vi "Get INFO from ini FILE - AMSClient.vi"(0 "ini Name":string="AMSClient.ini", 5 "Application Directory (Default if blank)":path, 11 "Error In":errorcluster) -> (1 "Settings":T3, 4 "ini Path":path=path "C:/Users/CK/workspace/LabVIEW/Configuration File Test/MyEXE.ini", 6 "Connection Information":T1={"Connection "="SQL Server 32bit HPEnvy", "Username"="admin", "Password"="admin123"}, 8 "AMS Connection Information":T1={"Connection "="SQL Server 32bit HPEnvy", "Username"="admin", "Password"="admin123"}, 10 "Settings Boolean":T2, 12 "MessageQ":string, 15 "Error Out":errorcluster)   [LabVIEW 2013]
uses:
  Controls/Connection Information Cluster.ctl
  <vilib>/Utility/config.llb/Read Key (String).vi
  <vilib>/Utility/config.llb/Read Key (Boolean).vi
  <vilib>/Utility/config.llb/NI_LVConfig.lvlib
  <vilib>/Utility/config.llb/Write Key (I32).vi
panel:
  out "Application Directory":path=path "C:/Users/CK/workspace/LabVIEW/Configuration File Test"
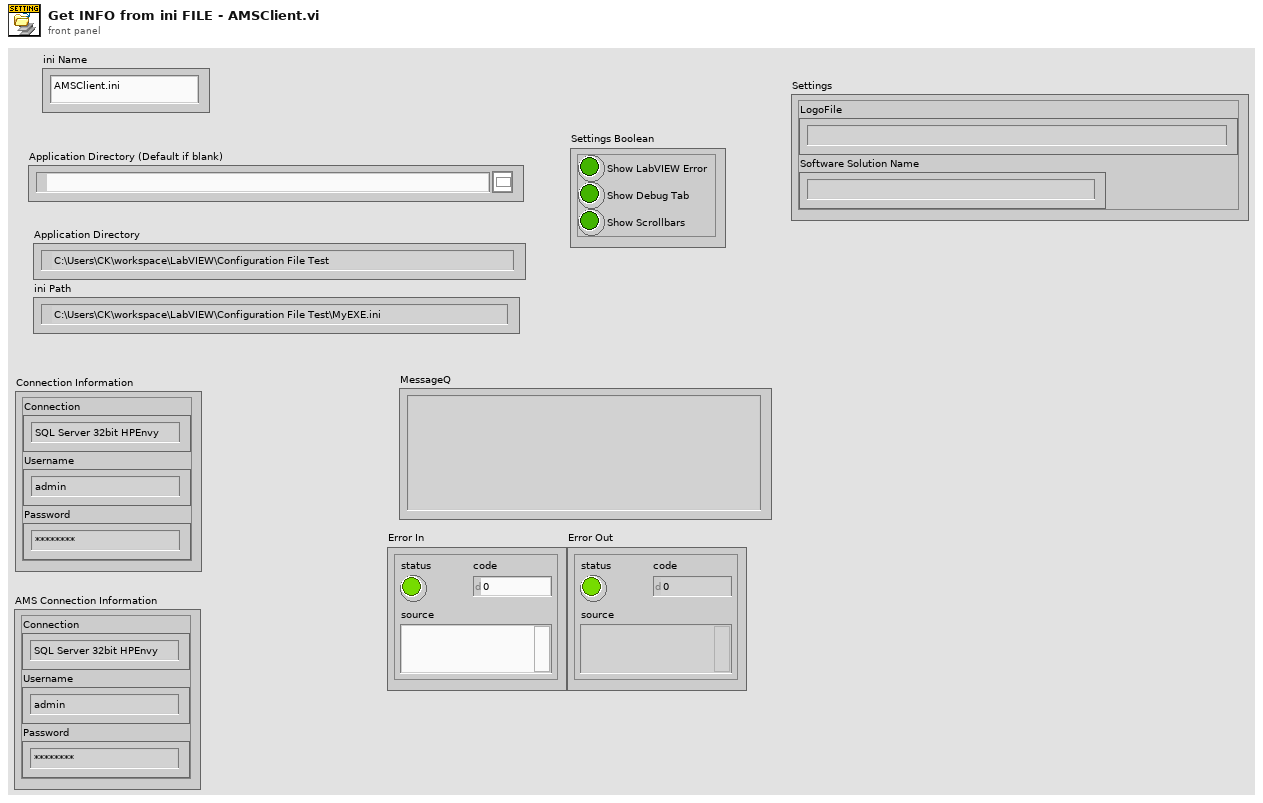
[diagram p1: front panel]
types:
  T1 = typedef "Connection Information Cluster.ctl" = cluster{"Connection ":string, "Username":string, "Password":string}
  T2 = cluster{"Show LabVIEW Error":bool, "Show Debug Tab":bool, "Show Scrollbars":bool}
  T3 = cluster{"LogoFile":string, "Software Solution Name":string}
  T4 = typedef "NI_LVConfig.lvlib/Config Data RefNum.ctl" = refnum<k1>
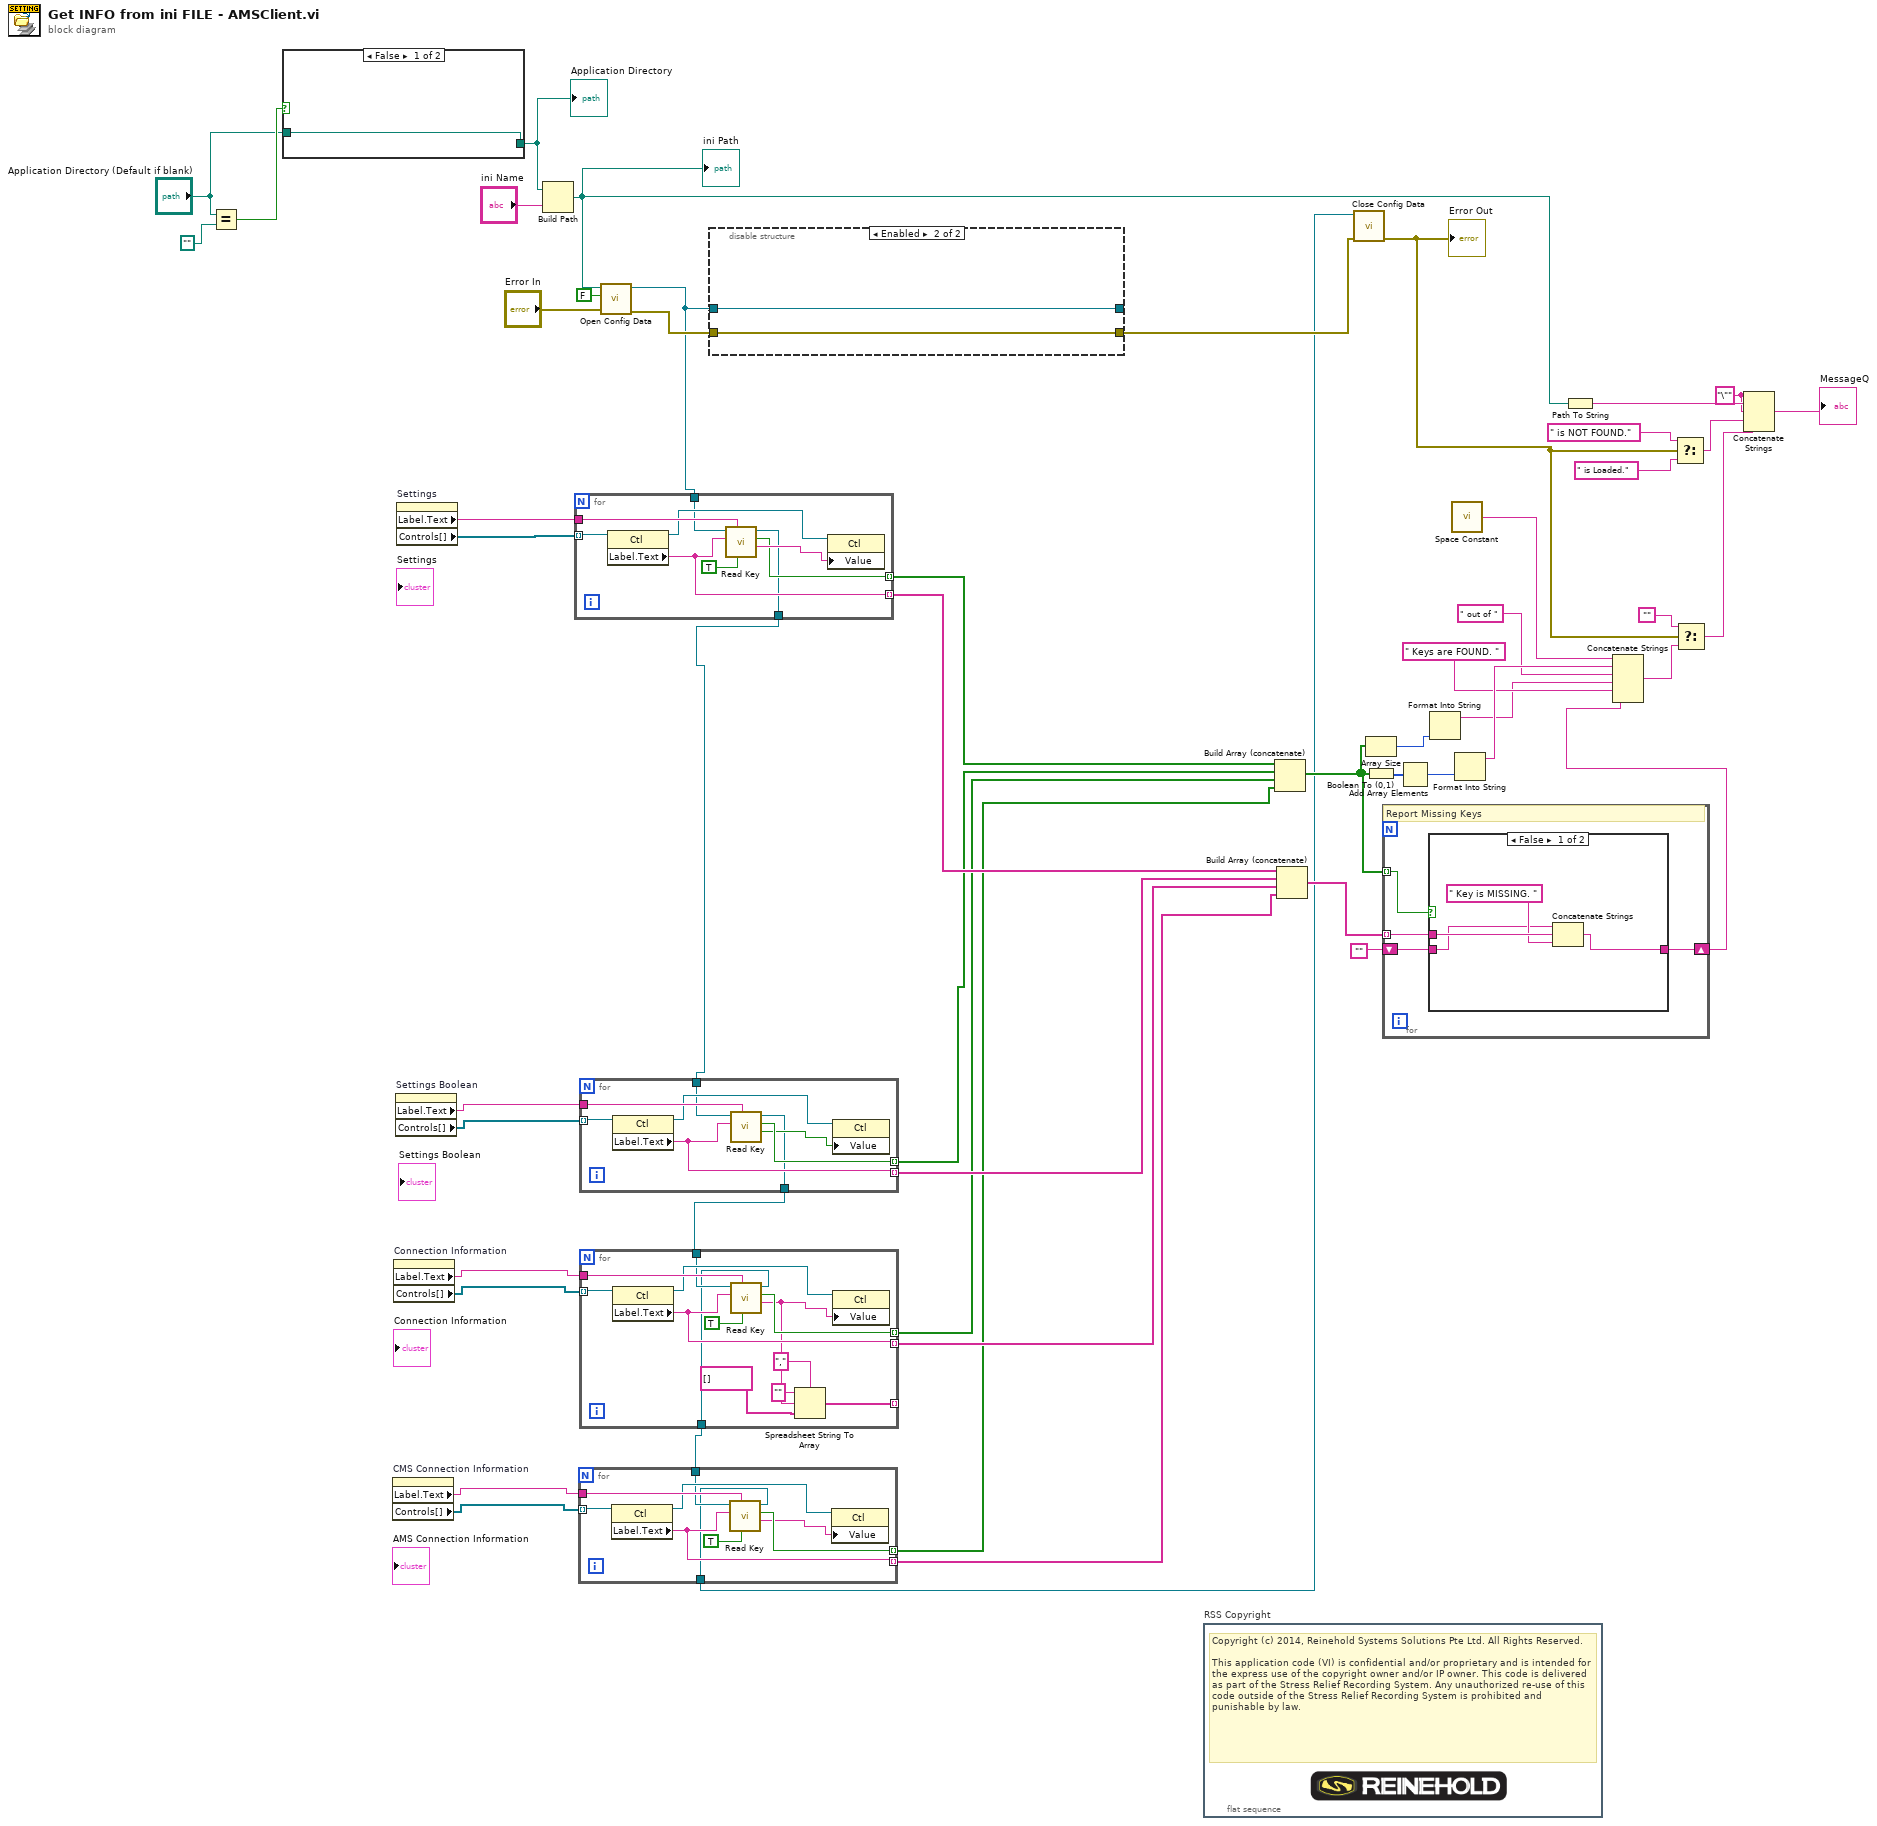
[diagram p0: block diagram]
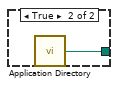
[diagram p2: hidden frame]
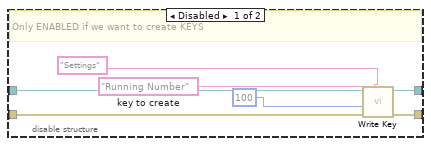
[diagram p4: hidden frame]
diagram:
  w47 = "\"" ("string")
  n1 = Equal?(x="Application Directory (Default if blank)", y=path "") -> (x = y?=w25:bool)
  n2 = case shown="False" w25 {
    tunnel: [w54 w55] -> w53
    tunnel: "Application Directory (Default if blank)" -> [w54 _]
    frame False {
    }
    frame True {
      n3 = call <vilib>:"Application Directory.vi"() -> ("Application Directory"=w55:path)
    }
  }
  "Application Directory" <- w53
  n4 = property on="CMS Connection Information" class="Clust (strict)"() -> ("Label.Text"=w6:string, "Controls[]"=w7:refnum<vi>[])  [unwired: 2 in, 2 out]
  n5 = property on="Connection Information" class="Clust (strict)"() -> ("Label.Text"=w11:string, "Controls[]"=w10:refnum<vi>[])  [unwired: 2 in, 2 out]
  n6 = property on="Settings Boolean" class="Clust (strict)"() -> ("Label.Text"=w13:string, "Controls[]"=w17:refnum<vi>[])  [unwired: 2 in, 2 out]
  n7 = property on="Settings" class="Clust (strict)"() -> ("Label.Text"=w21:string, "Controls[]"=w22:refnum<vi>[])  [unwired: 2 in, 2 out]
  n8 = Build Path(base path=w53, name or relative path="ini Name") -> (appended path=w49:path)
  "ini Path" <- w49
  n9 = call <vilib>:"Open Config Data.vi"("error in (no error)"="Error In", "create file if necessary (T)"=FALSE, "configuration file path"=w49) -> ("error out"=w50:errorcluster, "refnum"=w18:T4)  [unwired: 6 in, 1 out]
  n10 = for {
    tunnel: w22 -> [w64] mode=indexing
    tunnel: w21 -> [w63]
    tunnel: [w60] -> w20 mode=indexing
    tunnel: w18 -> [w59]
    tunnel: [w58] -> w19 mode=indexing
    tunnel: [w57] -> w1
    n11 = property class="Ctl"(reference=w64) -> (reference out=w62:refnum<vi>, "Label.Text"=w58:string)  [unwired: 1 in, 1 out]
    n12 = call-poly <vilib>:"Read Key.vi"("read raw string? (F)"=TRUE, "section"=w63, "key"=w58, "refnum"=w59) -> ("value"=w61:string, "found?"=w60:bool, "refnum out"=w57:T4)  [unwired: 4 in, 1 out]
    n13 = property class="Ctl"(reference=w62, "Value"=w61) -> ()  [unwired: 1 in, 2 out]
  }
  n14 = for {
    tunnel: w17 -> [w72] mode=indexing
    tunnel: w13 -> [w71]
    tunnel: [w69] -> w15 mode=indexing
    tunnel: w1 -> [w68]
    tunnel: [w67] -> w16 mode=indexing
    tunnel: [w65] -> w12
    n15 = property class="Ctl"(reference=w72) -> (reference out=w70:refnum<vi>, "Label.Text"=w67:string)  [unwired: 1 in, 1 out]
    n16 = call-poly <vilib>:"Read Key.vi"("section"=w71, "key"=w67, "refnum"=w68) -> ("value"=w66:bool, "found?"=w69:bool, "refnum out"=w65:T4)  [unwired: 5 in, 1 out]
    n17 = property class="Ctl"(reference=w70, "Value"=w66) -> ()  [unwired: 1 in, 2 out]
  }
  n18 = for {
    tunnel: w10 -> [w85] mode=indexing
    tunnel: w11 -> [w84]
    tunnel: [w82] -> w9 mode=indexing
    tunnel: w12 -> [w81]
    tunnel: [w80] -> w8 mode=indexing
    tunnel: [w75] -> _ mode=indexing
    tunnel: [w74] -> w5
    n19 = property class="Ctl"(reference=w85) -> (reference out=w83:refnum<vi>, "Label.Text"=w80:string)  [unwired: 1 in, 1 out]
    n20 = call-poly <vilib>:"Read Key.vi"("read raw string? (F)"=TRUE, "section"=w84, "key"=w80, "refnum"=w81) -> ("value"=w79:string, "found?"=w82:bool, "refnum out"=w74:T4)  [unwired: 4 in, 1 out]
    n21 = Spreadsheet String To Array(delimiter (Tab)=",", format string="", spreadsheet string=w79, array type (2D Dbl)=string[] []) -> (array=w75:string[])
    n22 = property class="Ctl"(reference=w83, "Value"=w79) -> ()  [unwired: 1 in, 2 out]
  }
  n23 = for {
    tunnel: w7 -> [w94] mode=indexing
    tunnel: w6 -> [w93]
    tunnel: [w91] -> w3 mode=indexing
    tunnel: w5 -> [w90]
    tunnel: [w89] -> w2 mode=indexing
    tunnel: [w87] -> w4
    n24 = property class="Ctl"(reference=w94) -> (reference out=w92:refnum<vi>, "Label.Text"=w89:string)  [unwired: 1 in, 1 out]
    n25 = call-poly <vilib>:"Read Key.vi"("read raw string? (F)"=TRUE, "section"=w93, "key"=w89, "refnum"=w90) -> ("value"=w88:string, "found?"=w91:bool, "refnum out"=w87:T4)  [unwired: 4 in, 1 out]
    n26 = property class="Ctl"(reference=w92, "Value"=w88) -> ()  [unwired: 1 in, 2 out]
  }
  n27 = disable-structure shown="Enabled" {
    disable-tunnel: w50 -> [w101 w102]
    disable-tunnel: [w98 w102] -> w14
    disable-tunnel: [w99 w103] -> _
    disable-tunnel: w18 -> [w100 w103]
    frame Disabled {
      w97 = "Running Number"  # key to create
      # "Only ENABLED if we want to create KEYS"
      n28 = call-poly <vilib>:"Write Key.vi"("section"="Settings", "error in (no error)"=w101, "value"=100 ("default value"), "key"=w97, "refnum"=w100) -> ("error out"=w98:errorcluster, "refnum out"=w99:T4)  [unwired: 4 in, 1 out]
    }
    frame Enabled {
    }
  }
  n29 = flat-sequence "RSS Copyright" {
    frame #0 {
      # "Copyright (c) 2014, Reinehold Systems Solutions Pte Ltd. All Rights Reserved.\n\nThis application code (VI) is confidential and/or proprietary and is intended for the express use of the copyright owner and/or IP owner. This code is delivered as part of the Stress Relief Recording System. Any unauthorized re-use of this code outside of the Stress Relief Recording System is prohibited and punishable by law."
    }
  }
  n30 = Build Array (concatenate)(w20, w15, w9, w3) -> (w29:bool[])
  n31 = Build Array (concatenate)(w19, w16, w8, w2) -> (w23:string[])
  n32 = call <vilib>:"Close Config Data.vi"("error in (no error)"=w14, "refnum"=w4) -> ("error out"=w33:errorcluster)  [unwired: 8 in, 1 out]
  "Error Out" <- w33
  n33 = Array Size(array=w29) -> (size(s)=w28:i32)
  n34 = Boolean To (0,1)(Boolean=w29) -> (0, 1=w42:i16[])
  n35 = for {
    tunnel: w29 -> [w107] mode=indexing
    tunnel: w23 -> [w106] mode=indexing
    shift-right: [w104] -> w31
    shift-left: "" -> [w105]
    # "Report Missing Keys"
    n36 = case shown="False" w107 {
      tunnel: w106 -> [w111 _]
      tunnel: w105 -> [w109 w112]
      tunnel: [w108 w112] -> w104
      frame False {
        n37 = Concatenate Strings(w109, w111, " Key is MISSING. " ("string")) -> (w108:string)
      }
      frame True {
      }
    }
  }
  n38 = Add Array Elements(numeric array=w42) -> (sum=w41:i16)
  n39 = Format Into String(w28) -> (resulting string=w27:string)  [unwired: 3 in, 1 out]
  n40 = call <vilib>:"Space Constant.vi"() -> ("String"=w39:string)
  n41 = Format Into String(w41) -> (resulting string=w38:string)  [unwired: 3 in, 1 out]
  n42 = Path To String(path=w49) -> (string=w48:string)
  n43 = Concatenate Strings(w39, w38, " out of " ("string"), w27, " Keys are FOUND. " ("string"), w31) -> (w36:string)
  n44 = Select(t=" is NOT FOUND." ("string"), s=w33, f=" is Loaded." ("string")) -> (s? t:f=w45:string)
  n45 = Select(t="", s=w33, f=w36) -> (s? t:f=w35:string)
  n46 = Concatenate Strings(w47, w48, w47, w45, w35) -> (→"MessageQ":string)
